vi "Mine Help Files.vi"() -> ()   [LabVIEW 2015]
doc: "<b> </b> <b> </b>\n©2016 Q Software Innovations, LLC (QSI)\nwritten by Quentin Alldredge\nproduced in LabVIEW 2015"
uses:
  Project Manipulation Scripts/Project Manipulation Scripts.lvlib
  VI Server Toolkit/Lookup Class by ID (String).vi
panel:
  out "Read Only Scripts":path[](array[path])
  out "Array":T1(array[cluster])
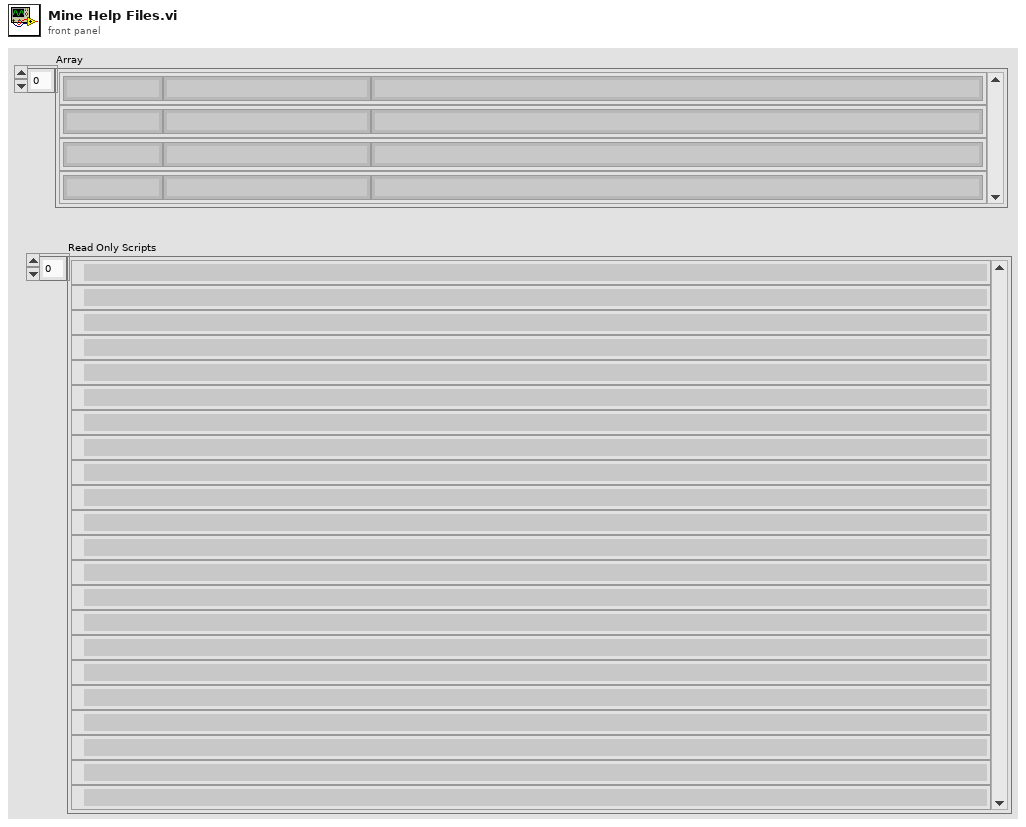
[diagram p1: front panel]
types:
  T1 = cluster{"Class Name (unlocalized)":string, "Long name (localized)":string, string}[]
  T2 = typedef "ASC_UniqueIDStringParentIDStringName.ctl" = cluster{"Unique ID string":string, "Parent ID string":string, "Class Name (unlocalized)":string, "Class Name (localized)":string}
  T3 = typedef "ASPM_UniqueIDStringDatanameShortnameLongname.ctl" = cluster{"Unique ID string":string, "Data name":string, "Short name (localized)":string, "Long name (localized)":string}
  T4 = typedef "VI Server Toolkit.lvlib/Property Flags.ctl" = cluster{"CanRead":bool, "CanWrite":bool, "IsDeprecated":bool, "IsPrivate":bool, "IsScripting":bool, "IsNotInRun-Time":bool}
  T5 = cluster{"Class Name (unlocalized)":string, "Long name (localized)":string, string}
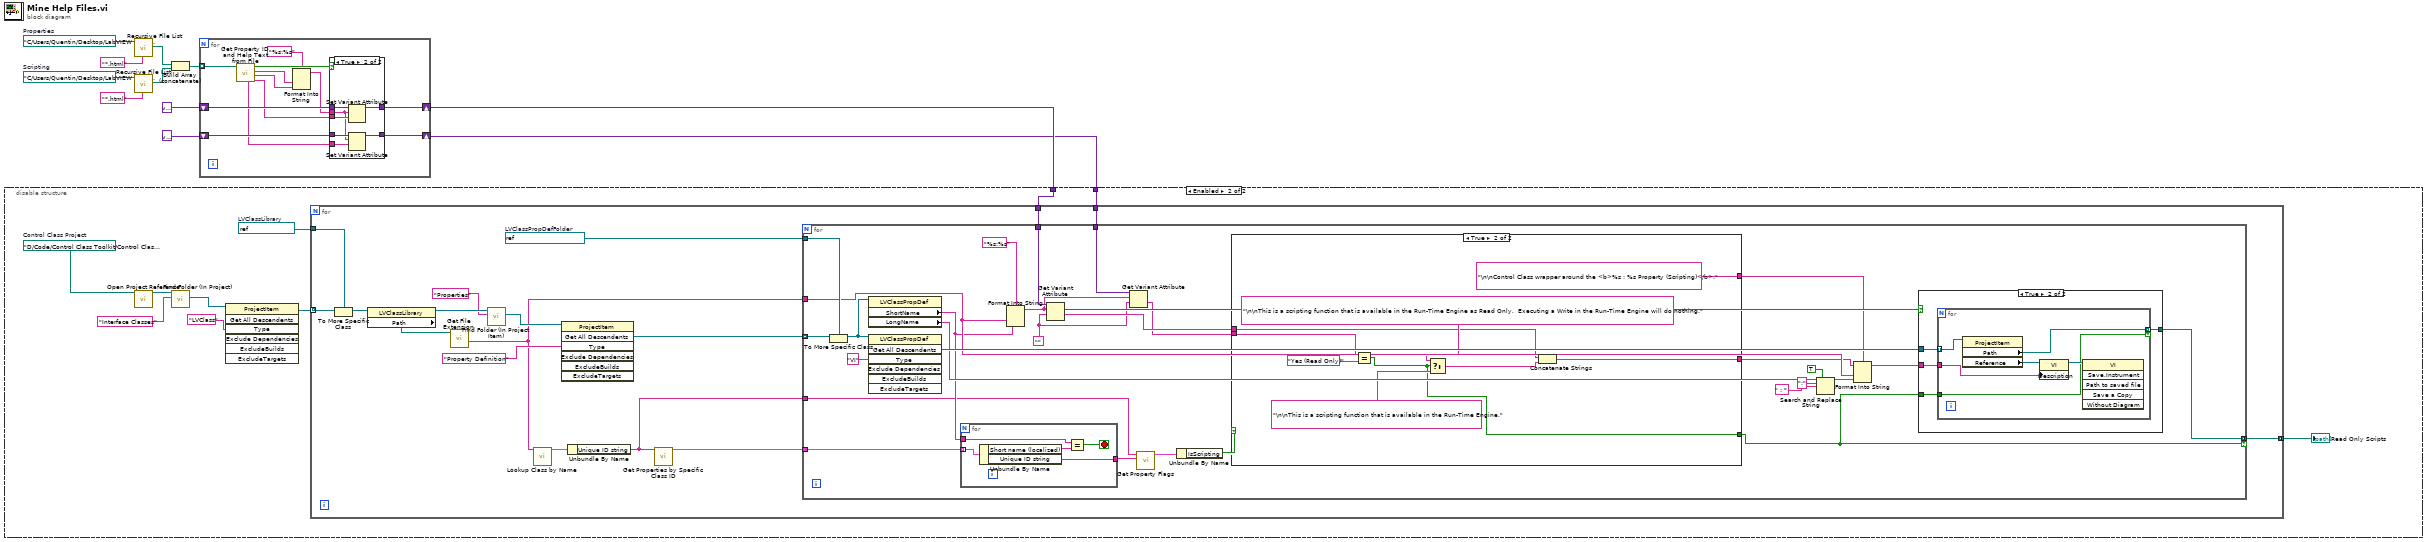
[diagram p0: block diagram]
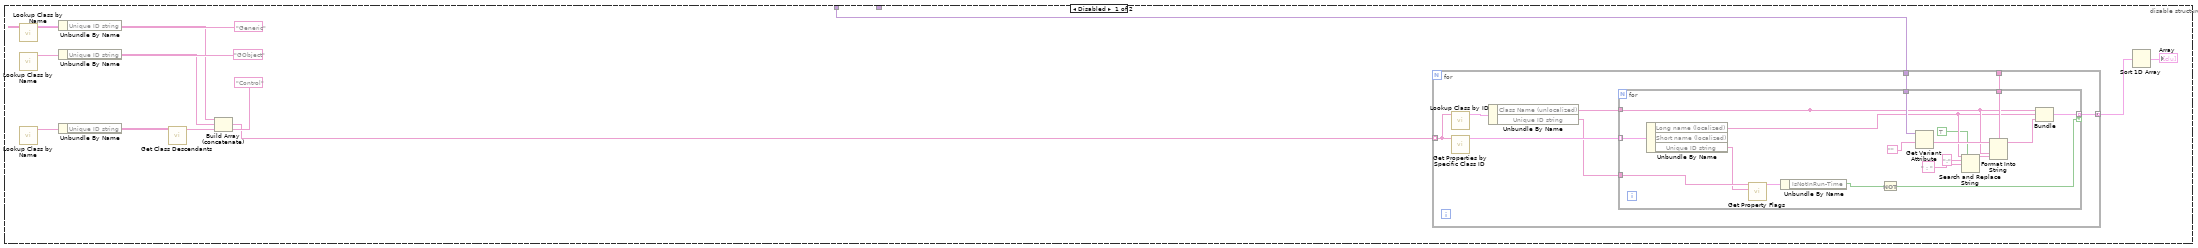
[diagram p2: hidden frame]
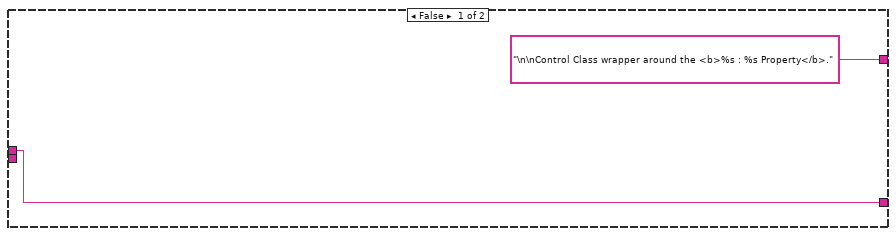
[diagram p3: hidden frame]
diagram:
  w10 = path "C:/Users/Quentin/Desktop/LabVIEW Help HTML/lvscript.chm"  # Scripting
  w11 = path "C:/Users/Quentin/Desktop/LabVIEW Help HTML/lvprop.chm"  # Properties
  n1 = call <vilib>:"Recursive File List.vi"("pattern"="*.html", "Folder Path"=w11) -> ("All Files in Dir"=w6:path[])  [unwired: 5 in, 4 out]
  n2 = call <vilib>:"Recursive File List.vi"("pattern"="*.html", "Folder Path"=w10) -> ("All Files in Dir"=w5:path[])  [unwired: 5 in, 4 out]
  n3 = Build Array (concatenate)(w6, w5) -> (w9:path[])
  n4 = for {
    tunnel: w9 -> [w23] mode=indexing
    shift-right: [w20] -> w3
    shift-left: variant -> [w22]
    shift-right: [w13] -> w1
    shift-left: variant -> [w14]
    n5 = call "Get Property ID and Help Text from File.vi"("Path"=w23) -> ("Context Help"=w15:string, "ShortName"=w17:string, "Class"=w19:string, "Found?"=w21:bool, "Available in Run-Time"=w12:string)  [unwired: 6 in]
    n6 = Format Into String(format string="%s:%s", w19, w17) -> (resulting string=w18:string)  [unwired: 2 in, 1 out]
    n7 = case shown="True" w21 {
      tunnel: w22 -> [w25 w32]
      tunnel: w18 -> [_ w27]
      tunnel: w15 -> [_ w31]
      tunnel: [w25 w30] -> w20
      tunnel: w14 -> [w24 w29]
      tunnel: [w24 w28] -> w13
      tunnel: w12 -> [_ w26]
      frame False {
      }
      frame True {
        n8 = Set Variant Attribute(Variant=w32, name=w27, value=w31) -> (Variant out=w30:variant)  [unwired: 1 in, 2 out]
        n9 = Set Variant Attribute(Variant=w29, name=w27, value=w26) -> (Variant out=w28:variant)  [unwired: 1 in, 2 out]
      }
    }
  }
  n10 = disable-structure shown="Enabled" {
    disable-tunnel: w3 -> [w43 w78]
    disable-tunnel: w1 -> [_ w77]
    frame Disabled {
      n11 = call "Lookup Class by Name.vi"("Class Name"="Generic") -> ("Class Information"=w39:T2)  [unwired: 8 in, 2 out]
      n12 = call "Lookup Class by Name.vi"("Class Name"="GObject") -> ("Class Information"=w37:T2)  [unwired: 8 in, 2 out]
      n13 = call "Lookup Class by Name.vi"("Class Name"="Control") -> ("Class Information"=w46:T2)  [unwired: 8 in, 2 out]
      n14 = Unbundle By Name(w39) -> ("Unique ID string"=w38:string)
      n15 = Unbundle By Name(w37) -> ("Unique ID string"=w36:string)
      n16 = Unbundle By Name(w46) -> ("Unique ID string"=w45:string)
      n17 = call "Get Class Descendants.vi"("Class ID"=w45) -> ("Class Descendant IDs[]"=w44:string[])  [unwired: 9 in, 1 out]
      n18 = Build Array (concatenate)(w38, w36, w44) -> (w40:string[])
      n19 = for {
        tunnel: w40 -> [w53] mode=indexing
        tunnel: w43 -> [w54]
        tunnel: [w50] -> w34 mode=concatenating
        tunnel: [w48] -> w35
        n20 = call-poly "Lookup Class by ID.vi"("Class ID"=w53) -> ("Class Information"=w52:T2)  [unwired: 8 in, 2 out]
        n21 = call "Get Properties by Specific Class ID.vi"("Class ID"=w53) -> ("Properties[]"=w55:T3[])  [unwired: 10 in]
        n22 = Unbundle By Name(w52) -> ("Class Name (unlocalized)"=w51:string, "Unique ID string"=w49:string)
        n23 = for {
          tunnel: w55 -> [w75] mode=indexing
          tunnel: w54 -> [w74]
          tunnel: w51 -> [w62]
          tunnel: [w72] -> w50 mode=indexing if=w65
          tunnel: w49 -> [w69]
          tunnel: w48 -> [w63]
          n24 = Unbundle By Name(w75) -> ("Long name (localized)"=w60:string, "Short name (localized)"=w71:string, "Unique ID string"=w68:string)
          n25 = call "Get Property Flags.vi"("Property ID"=w68, "Class ID"=w69) -> ("Property Flags"=w67:T4)  [unwired: 8 in, 1 out]
          n26 = Unbundle By Name(w67) -> ("IsNotInRun-Time"=w66:bool)
          n27 = Not(x=w66) -> (.not. x?=w65:bool)
          n28 = Get Variant Attribute(Variant=w74, default value (empty Variant)="") -> (name=w70:string, value=w64:string)  [unwired: 1 in, 3 out]
          n29 = Search and Replace String(replace all?=TRUE ("replace all? (F)"), input string=w60, search string=":", replace string=" : " ("replace string (\"\")")) -> (result string=w59:string)  [unwired: 4 in, 3 out]
          n30 = Format Into String(format string=w63, initial string=w64, w62, w59) -> (resulting string=w61:string)  [unwired: 1 in, 1 out]
          n31 = Bundle("Class Name (unlocalized)"=w62, "Long name (localized)"=w60, w61) -> (w72:T5)  [unwired: 1 in]
        }
      }
      n32 = Sort 1D Array(array=w34) -> (sorted array=→"Array":T1)
    }
    frame Enabled {
      w79 = refnum<vi> refnum  # LVClassLibrary
      w85 = path "D:/Code/Control Class Toolkit/Control Class Toolkit.lvproj"  # Control Class Project
      n33 = call "Open Project Reference.vi"("Project Path"=w85) -> ("Project out"=w84:refnum<vi>)  [unwired: 10 in]
      n34 = call "Find Folder (In Project).vi"("Folder Name"="Interface Classes", "Project in"=w84) -> ("Folder Refnum"=w82:refnum<vi>)  [unwired: 7 in, 2 out]
      n35 = invoke class="ProjectItem" method="Get All Descendents"(reference=w82, "Type"="LVClass") -> ("All Descendents"=w80:refnum<vi>[])  [unwired: 5 in, 6 out]
      n36 = for {
        tunnel: w80 -> [w102] mode=indexing
        tunnel: w79 -> [w94]
        tunnel: w78 -> [w92]
        tunnel: w77 -> [w87]
        tunnel: [w86] -> w76 mode=concatenating
        w93 = refnum<vi> refnum  # LVClassPropDefFolder
        n37 = To More Specific Class(target class=w94, reference=w102) -> (specific class reference=w95:refnum<vi>)  [unwired: 1 in, 1 out]
        n38 = property class="LVClassLibrary"(reference=w95) -> (reference out=w100:refnum<vi>, "Path"=w101:path)  [unwired: 1 in, 1 out]
        n39 = call <vilib>:"Get File Extension.vi"("file"=w101) -> ("filename without extension"=w91:string)  [unwired: 6 in, 4 out]
        n40 = call "Find Folder (In Project Item).vi"("Folder Name"="Properties", "ProjectItem in"=w100) -> ("Folder Refnum"=w98:refnum<vi>)  [unwired: 7 in, 2 out]
        n41 = call "Lookup Class by Name.vi"("Class Name"=w91) -> ("Class Information"=w90:T2)  [unwired: 8 in, 2 out]
        n42 = invoke class="ProjectItem" method="Get All Descendents"(reference=w98, "Type"="Property Definition") -> ("All Descendents"=w96:refnum<vi>[])  [unwired: 5 in, 6 out]
        n43 = Unbundle By Name(w90) -> ("Unique ID string"=w88:string)
        n44 = call "Get Properties by Specific Class ID.vi"("Class ID"=w88) -> ("Properties[]"=w89:T3[])  [unwired: 10 in]
        n45 = for {
          tunnel: w96 -> [w132] mode=indexing
          tunnel: w93 -> [w129]
          tunnel: w91 -> [w121]
          tunnel: w92 -> [w126]
          tunnel: w89 -> [w118]
          tunnel: w88 -> [w116]
          tunnel: w87 -> [w109]
          tunnel: [w103] -> w86 mode=concatenating if=w104
          w107 = ""
          n46 = To More Specific Class(target class=w129, reference=w132) -> (specific class reference=w128:refnum<vi>)  [unwired: 1 in, 1 out]
          n47 = property class="LVClassPropDef"(reference=w128) -> ("ShortName"=w117:string, "LongName"=w119:string)  [unwired: 1 in, 2 out]
          n48 = invoke class="LVClassPropDef" method="Get All Descendents"(reference=w128, "Type"="VI") -> ("All Descendents"=w130:refnum<vi>[])  [unwired: 5 in, 6 out]
          n49 = for {
            tunnel: w118 -> [w148] mode=indexing
            tunnel: w117 -> [w146]
            tunnel: [w144] -> w115
            stop <- w145 stop-if-true
            n50 = Unbundle By Name(w148) -> ("Short name (localized)"=w147:string, "Unique ID string"=w144:string)
            n51 = Equal?(x=w146, y=w147) -> (x = y?=w145:bool)
          }
          n52 = Format Into String(format string="%s:%s", w121, w117) -> (resulting string=w108:string)  [unwired: 2 in, 1 out]
          n53 = Get Variant Attribute(Variant=w126, name=w108, default value (empty Variant)=w107) -> (found=w125:bool, value=w110:string)  [unwired: 1 in, 2 out]
          n54 = Get Variant Attribute(Variant=w109, name=w108, default value (empty Variant)=w107) -> (value=w106:string)  [unwired: 1 in, 3 out]
          n55 = call "Get Property Flags.vi"("Property ID"=w115, "Class ID"=w116) -> ("Property Flags"=w114:T4)  [unwired: 8 in, 1 out]
          n56 = Unbundle By Name(w114) -> ("IsScripting"=w113:bool)
          n57 = case shown="True" w113 {
            tunnel: w106 -> [_ w143]
            tunnel: w110 -> [w134 w139]
            tunnel: [w134 w137] -> w112
            tunnel: [_ w136] -> w104
            tunnel: ["\n\nControl Class wrapper around the <b>%s : %s Property</b>." ("format string") "\n\nControl Class wrapper around the <b>%s : %s Property (Scripting)</b>." ("format string")] -> w105
            frame False {
            }
            frame True {
              n58 = Equal?(x=w143, y="Yes (Read Only)") -> (x = y?=w136:bool)
              n59 = Select(t="\n\nThis is a scripting function that is available in the Run-Time Engine as Read Only.  Executing a Write in the Run-Time Engine will do nothing." ("format string"), s=w136, f="\n\nThis is a scripting function that is available in the Run-Time Engine." ("format string")) -> (s? t:f=w138:string)
              n60 = Concatenate Strings(w139, w138) -> (w137:string)
            }
          }
          n61 = Search and Replace String(replace all?=TRUE ("replace all? (F)"), input string=w119, search string=":", replace string=" : " ("replace string (\"\")")) -> (result string=w124:string)  [unwired: 4 in, 3 out]
          n62 = Format Into String(format string=w105, initial string=w112, w121, w124) -> (resulting string=w111:string)  [unwired: 1 in, 1 out]
          n63 = case shown="True" w125 {
            tunnel: w130 -> [_ w152]
            tunnel: w111 -> [_ w151]
            tunnel: w104 -> [_ w150]
            tunnel: [_ w149] -> w103
            frame False {
            }
            frame True {
              n64 = for {
                tunnel: w152 -> [w158] mode=indexing
                tunnel: w151 -> [w156]
                tunnel: w150 -> [w153]
                tunnel: [w154] -> w149 mode=indexing if=w153
                n65 = property class="ProjectItem"(reference=w158) -> ("Path"=w154:path, "Reference"=w157:refnum<vi>)  [unwired: 1 in, 2 out]
                n66 = property class="VI"(reference=w157, "Description"=w156) -> (reference out=w155:refnum<vi>)  [unwired: 1 in, 1 out]
                n67 = invoke class="VI" method="Save.Instrument"(reference=w155) -> ()  [unwired: 5 in, 6 out]
              }
            }
          }
        }
      }
      "Read Only Scripts" <- w76
    }
  }
